vi "Read Batch Profiles(for Advanced Mode).vi"(0 "Device ID (0)":i32, 5 "Read Req":T5 {"Batch Pos" items=["CURRENT", "SPECIFY", "COMMITED", "NEWEST PROFILE"]}, 9 "Data Size (0: Auto Size)":u32, 11 "error in (no error)":errorcluster) -> (3 "Profile Info":T7, 4 "Device ID out":i32, 6 "Batch Data":u32[](array[numeric]), 8 "Profile Rsp":T4, 10 "Batch Measure Data":T1[](array[typedef]) {"Judge Result" items=["HI", "GO", "LO", "ALARM"]; "Data Info" items=["VALID", "ALARM", "WAIT"]}, 14 "Measure Data":T1[](array[typedef]) {"Judge Result" items=["HI", "GO", "LO", "ALARM"]; "Data Info" items=["VALID", "ALARM", "WAIT"]}, 15 "error out":errorcluster)   [LabVIEW 8.6, in "Keyence LJ-V7000.lvlib"]
doc: "This function gets profile data.\nProfile data is stored in 0.01 μm units.\n\n<B>Note</B>:\nFor the details on the data stored in the profile data (storage order and size), refer to <B>10.3</B> in a manual of measuring instrument drivers.\n\nIf Compression(timse axis) is ON, use <B>Read Profiles(for Advanced Mode)</B> VI.\n\nTo read all of the profiles in one batch, read them with the procedure below.\n1. Call this VI by specifying <B>Current</B> for <B>Batch Pos</B> in <B>Read Req</B>. Save the start position and the amount of profiles that were read and the batch number that was read.\n2. Configure <B>Read Req</B> as listed below and call this VI again.\n　・<B>Batch Pos</B> = SPECIFY\n　・<B>Read Batch No</B> = batch number that was read\n　・<B>Read Profile Cnt</B> = starting profile number of the unread profiles in the batch\n3. Update <B>Read Profile Cnt</B> in step 2 and call this VI until all of the profiles in the batch can be read.\n\nWhen calling this VI, do not perform communication between the target controller and LJ-Navigation 2."
uses:
  Keyence LJ-V7000.lvlib
  constant/Driver VI No.ctl
  Clusters/Profile Info.ctl
  Clusters/Read Batch Profile Advance Rsp.ctl
  Private/vi/Low Level/Make VI Param(Read Batch Profile Advance Rsp).vi
  Private/vi/Low Level/Make DLL Param(Read Batch Profile Advance Req).vi
  Private/vi/Low Level/Make DLL Param(Read Batch Profile Advance Rsp).vi
  constant/Judge Result.ctl
  constant/Measure Data Info.ctl
  Clusters/Measure Data.ctl
  constant/Batch Pos.ctl
  Clusters/Read Batch Profile Advance Req.ctl
panel:
  # "(c) 2012 KEYENCE CORPORATION.  ALL RIGHTS RESERVED."
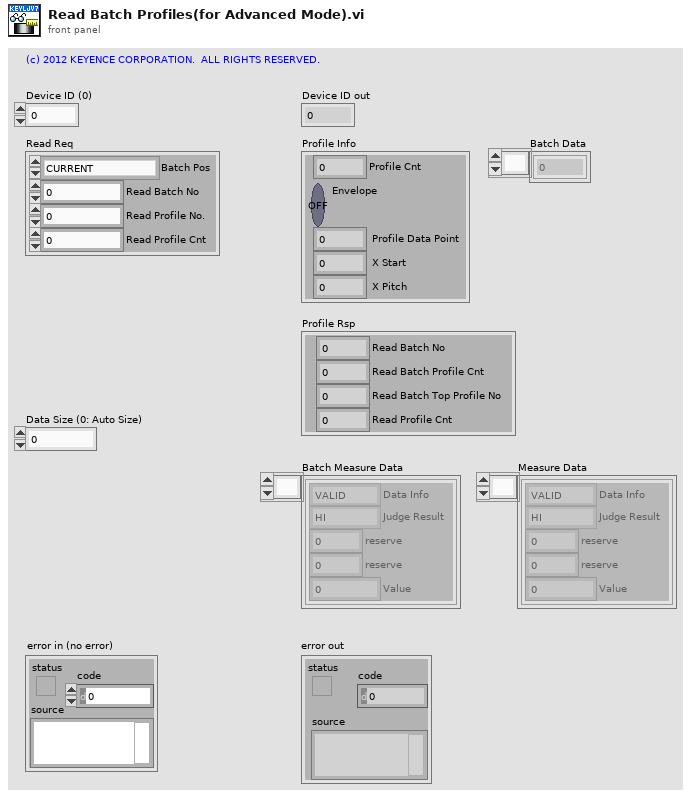
[diagram p1: front panel]
types:
  T1 = typedef "Keyence LJ-V7000.lvlib/Measure Data.ctl" = cluster{"Data Info":T2, "Judge Result":T3, "reserve":u8, "reserve":u8, "Value":sgl}
  T2 = typedef "Keyence LJ-V7000.lvlib/Measure Data Info.ctl" = u8
  T3 = typedef "Keyence LJ-V7000.lvlib/Judge Result.ctl" = u8
  T4 = typedef "Keyence LJ-V7000.lvlib/Read Batch Profile Advance Rsp.ctl" = cluster{"Read Batch No":u32, "Read Batch Profile Cnt":u32, "Read Batch Top Profile No":u32, "Read Profile Cnt":u8}
  T5 = typedef "Keyence LJ-V7000.lvlib/Read Batch Profile Advance Req.ctl" = cluster{"Batch Pos":T6, "Read Batch No":u32, "Read Profile No.":u32, "Read Profile Cnt":u8}
  T6 = typedef "Keyence LJ-V7000.lvlib/Batch Pos.ctl" = u8
  T7 = typedef "Keyence LJ-V7000.lvlib/Profile Info.ctl" = cluster{"Profile Cnt":u8, "Envelope":bool, " Profile Data Point":u16, " X Start":i32, " X Pitch":i32}
  T8 = typedef "Keyence LJ-V7000.lvlib/Driver VI No.ctl" = enum16{"Initialize", "Close", "Reboot Controller", "Return to Factory State", "Get System Error", "Clear System Error", "Trigger", "Start Batch Measurements", "Stop Batch Measurements", "Auto Zero", "Timing", "Reset", "Clear Memory", "Set Setting", "Get Setting", "Initialize Setting", "Reflect Setting", "Update Write Settings Area", "Check Status of Saving to Save Area", "Set Time", "Get Time", "Change Program", "Read Active Program Number", "Read Measurement Data", "Read Profiles(for High-Speed Mode)", "Read Batch Profiles(for High-Speed Mode)", "Read Profiles(for Advanced Mode)", "Read Batch Profiles(for Advanced Mode)", "Start Storage", "Stop Storage", "Read Storage Status", "Read Data Storage Data", "Read Profile Storage Data", "Read Batch Profile Storage Data", "Start High-Speed Data Communication", "Stop High-Speed Data Communication", "Read Profiles(for High-Speed Communication)"}
  T9 = cluster{"Batch Pos":T6, "reserve":u8, "reserve":u8, "reserve":u8, "Read Batch No":u32, "Read Profile No.":u32, "Read Profile Cnt":u8, "reserve":u8, "reserve":u8, "reserve":u8}
  T10 = cluster{"Read Batch No":u32, "Read Batch Profile Cnt":u32, "Read Batch Top Profile No":u32, "Read Profile Cnt":u8, "reserve":u8, "reserve":u8, "reserve":u8}
  T11 = cluster{"Profile Cnt":u8, u8, "reserve":u8, "reserve":u8, " Profile Data Point":u16, "reserve":u8, "reserve":u8, " X Start":i32, " XPitch":i32}
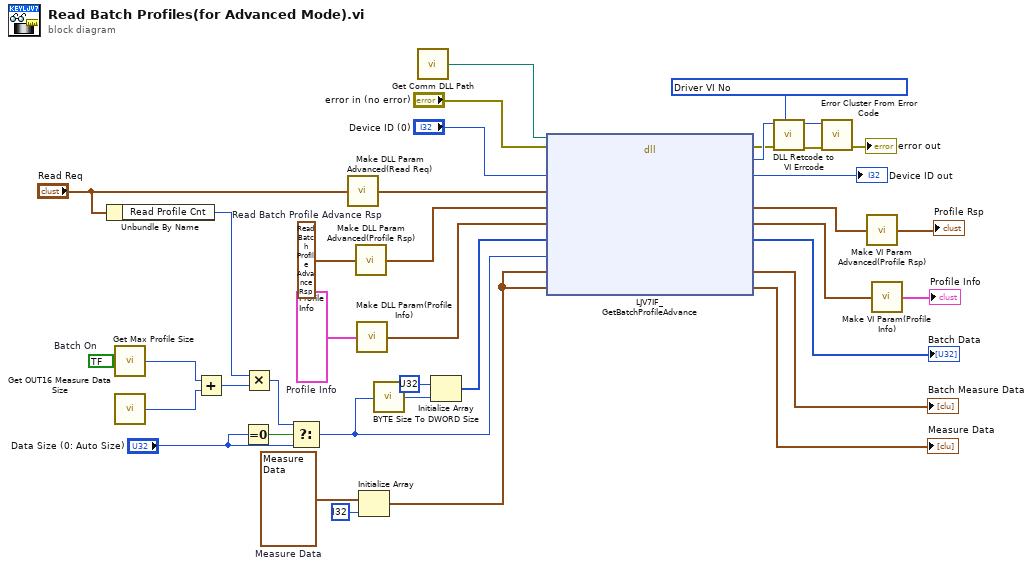
[diagram p0: block diagram]
diagram:
  w12 = bool ?  # Batch On
  w25 = T1 ?  # Measure Data
  w28 = T4 ?  # Read Batch Profile Advance Rsp
  w33 = T7 ?  # Profile Info
  n1 = Unbundle By Name("Read Req") -> ("Read Profile Cnt"=w4:u8)
  n2 = call "Get Max Profile Size.vi"("Batch On-Off"=w12) -> ("Profile Size"=w3:u32)  [unwired: 4 in]
  n3 = call "Get OUT16 Measure Data Size.vi"() -> ("OUT16 Measure Data Size"=w2:u32)  [unwired: 1 in]
  n4 = Add(x=w3, y=w2) -> (x+y=w1:u32)
  n5 = Equal To 0?(x="Data Size (0: Auto Size)") -> (x = 0?=w13:bool)
  n6 = Multiply(x=w4, y=w1) -> (x*y=w11:u32)
  n7 = Select(t=w11, s=w13, f="Data Size (0: Auto Size)") -> (s? t:f=w7:u32)
  n8 = call-poly "Make DLL Param Advanced(Read Req).vi"("Read Batch Profile Advance Req"="Read Req") -> ("pReq"=w30:T9)
  n9 = call-poly "Make DLL Param Advanced(Profile Rsp).vi"("Read Batch Profile Advance Rsp"=w28) -> ("pRsp"=w29:T10)
  n10 = call "Make DLL Param(Profile Info).vi"("Profile Info"=w33) -> ("DLL Parameter"=w32:T11)
  n11 = Initialize Array(w25, i32 ? ("次元サイズ")) -> (w23:T1[])
  n12 = call "BYTE Size To DWORD Size.vi"("BYTE Size"=w7) -> ("DWORD Size"=w10:u32)
  n13 = call "Get Comm DLL Path.vi"() -> ("Comm DLL Path"=w36:path)  [unwired: 1 in]
  n14 = Initialize Array(u32 ?, w10) -> (w9:u32[])
  n15 = dll-call lib="C:/Program Files/National Instruments/LabVIEW 2011/instr.lib/Keyence LJ-V7000/LJV7_IF.*" fn="LJV7IF_GetBatchProfileAdvance"(path in=w36, error in="error in (no error)", "lDeviceId"="Device ID (0)", "pReq"=w30, "pRsp"=w29, "pProfileInfo"=w32, "pdwProfileData"=w9, "dwDataSize"=w7, "pBatchMeasureData"=w23, "pMeasureData"=w23) -> (error out=w16:errorcluster, "lRetCode"=w17:i32, "lDeviceId"=→"Device ID out":i32, "pRsp"=w27:T10, "pProfileInfo"=w22:T11, "pdwProfileData"=→"Batch Data":u32[], "pBatchMeasureData"=→"Batch Measure Data":T1[], "pMeasureData"=→"Measure Data":T1[])  [unwired: 3 in, 1 out]
  n16 = call "DLL Retcode to VI Errcode.vi"("Driver VI No"=T8 ?, "error in (no error)"=w16, "DLL Return Code"=w17) -> ("error out"=w19:errorcluster, "VI Error Code"=w18:i32)  [unwired: 7 in]
  n17 = call <vilib>:"Error Cluster From Error Code.vi"("error in (no error)"=w19, "error code (0)"=w18) -> ("error out"=→"error out":errorcluster)  [unwired: 7 in]
  n18 = call-poly "Make VI Param Advanced(Profile Rsp).vi"("pRsp"=w27) -> ("Read Batch Profile Advance Rsp"=→"Profile Rsp":T4)
  n19 = call "Make VI Param(Profile Info).vi"("pProfileInfo"=w22) -> ("Profile Info"=→"Profile Info":T7)
